vi "Read NewTest.vi"(8 "error in (no error)":errorcluster, 11 "Assert Event in":refnum<class "Assert Event.lvclass">) -> (0 "error out":errorcluster, 2 "NewTest":T1(array[cluster]), 3 "Assert Event out":refnum<class "Assert Event.lvclass">)   [LabVIEW 2019, in "Assert.lvlib" / "Assert Event.lvclass"]
uses:
  Assert Event.lvclass
  Assert Event.lvclass/Assert Event.ctl
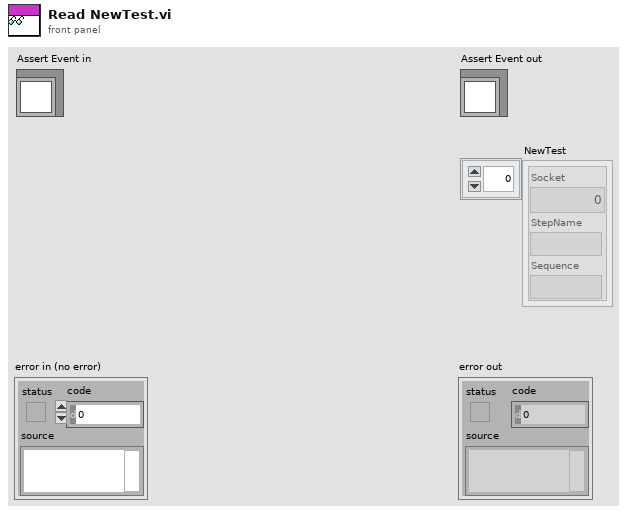
[diagram p1: front panel]
types:
  T1 = cluster{"Socket":i32, "StepName":string, "Sequence":string}[]
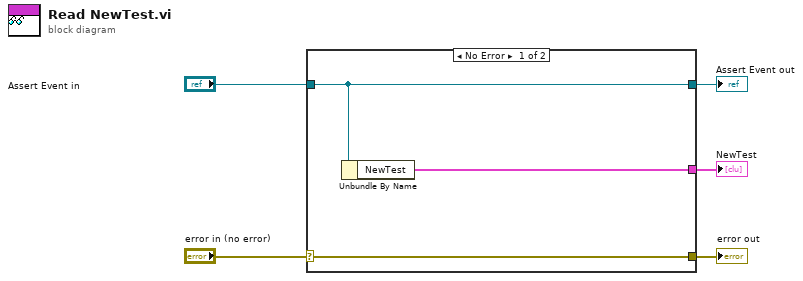
[diagram p0: block diagram]
diagram:
  n1 = case shown="No Error" "error in (no error)" {
    selector: "error in (no error)" -> [w8 w9]
    tunnel: [w8 w9] -> w4
    tunnel: [w7 w10] -> w2
    tunnel: "Assert Event in" -> [w7 w10]
    tunnel: [w6 _] -> w1
    frame No Error {
      n2 = Unbundle By Name(w7) -> ("NewTest"=w6:T1)
    }
    frame Error {
    }
  }
  "error out" <- w4
  "Assert Event out" <- w2
  "NewTest" <- w1
